vi "Stop.vi"(8 "Error In":errorcluster, 11 "Communicator in":refnum<class "Communicator.lvclass">) -> (0 "Error Out":errorcluster, 3 "Communicator out":refnum<class "Communicator.lvclass">)   [LabVIEW 2024, in "Communicator.lvclass"]
uses:
  Communicator.lvclass
  Communicator.lvclass/Communicator.ctl
  Interfaces/IRunnable/IRunnable.lvclass
  <vilib>/ActorFramework/Stop Msg/Stop Msg.lvclass
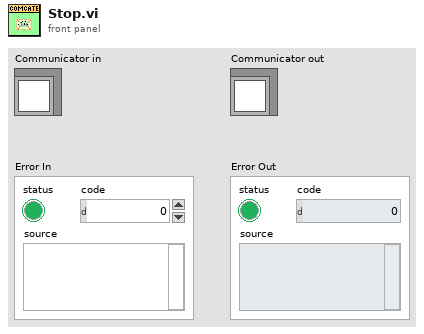
[diagram p1: front panel]
types:
  T1 = typedef "Communicator.lvclass/ObjectAttributes.ctl" = cluster{"IConfigure":refnum<class "IConfigure.lvclass">, "Worker Enqueuer":refnum<class "Message Enqueuer.lvclass">}
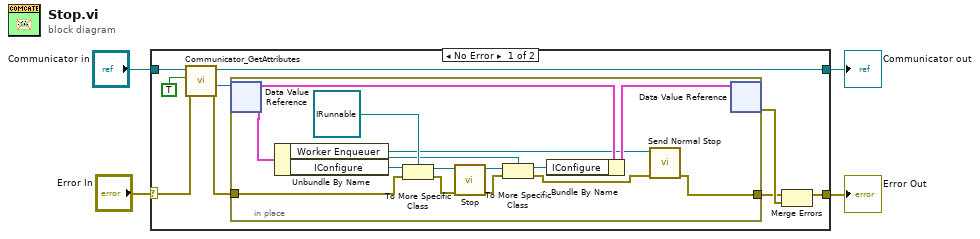
[diagram p0: block diagram]
diagram:
  n1 = case shown="No Error" "Error In" {
    selector: "Error In" -> [w13 w27]
    tunnel: [w12 w27] -> w3
    tunnel: "Communicator in" -> [w11 w28]
    tunnel: [w10 w28] -> w1
    frame No Error {
      n2 = call "Communicator_GetAttributes.vi"("Error In"=w13, "OnlyGetDvrReference(False)"=TRUE, "Communicator in"=w11) -> ("Error Out"=w6:errorcluster, "DataRef"=w8:refnum<data-value>, "Communicator out"=w10:refnum<class "Communicator.lvclass">)  [unwired: 5 in, 1 out]
      n3 = in-place {
        in-place-border: [w14] -> w5
        in-place-border: w6 -> [w17]
        n4 = in-place-dvr #1(w8) -> (w25:T1)  [unwired: 1 out]
        n5 = Unbundle By Name(w25) -> ("Worker Enqueuer"=w16:refnum<class "Message Enqueuer.lvclass">, "IConfigure"=w18:refnum<class "IConfigure.lvclass">)
        n6 = To More Specific Class(target class=refnum<class "IRunnable.lvclass"> refnum ("IRunnable.lvclass"), reference=w18, error in=w17) -> (specific class reference=w21:refnum<class "IRunnable.lvclass">, error out=w22:errorcluster)
        n7 = call-dynamic "Stop.vi"("error in"=w22, "IRunnable in"=w21) -> ("error out"=w20:errorcluster, "IRunnable out"=w19:refnum<class "IRunnable.lvclass">)  [unwired: 8 in]
        n8 = To More Specific Class(target class=w18, reference=w19, error in=w20) -> (specific class reference=w23:refnum<class "IConfigure.lvclass">, error out=w15:errorcluster)
        n9 = Bundle By Name(cluster=w25, "IConfigure"=w23) -> (w26:T1)
        n10 = call <vilib>:"Send Normal Stop.vi"("error in (no error)"=w15, "Message Enqueuer"=w16) -> ("error out"=w14:errorcluster)  [unwired: 9 in]
        n11 = in-place-dvr #1(w26) -> (w9:errorcluster)  [unwired: 1 out]
      }
      n12 = Merge Errors(w5, w9) -> (w12:errorcluster)
    }
    frame Error {
    }
  }
  "Error Out" <- w3
  "Communicator out" <- w1
